vi "DataEmulator.vi"(1 "Time":u32, 2 "queue out":refnum<queue>) -> ()   [LabVIEW 2018]
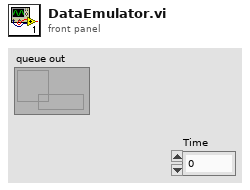
[diagram p1: front panel]
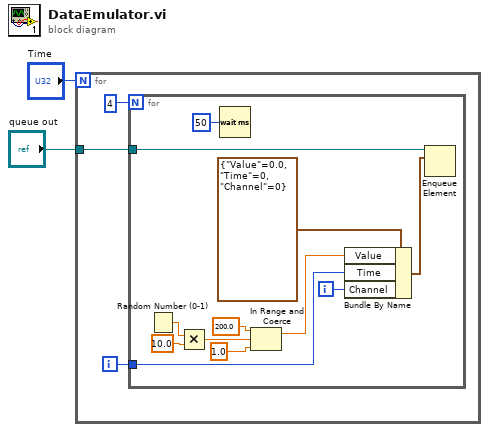
[diagram p0: block diagram]
diagram:
  n1 = for {
    N: "Time" -> [_]
    tunnel: "queue out" -> [w5]
    i -> [w4]
    n2 = for {
      N: 4 -> [_]
      tunnel: w5 -> [w17]
      tunnel: w4 -> [w7]
      i -> [w8]
      n3 = Random Number (0-1)() -> (number: 0 to 1=w16:dbl)
      n4 = Multiply(x=w16, y=10.0) -> (x*y=w14:dbl)
      n5 = Wait (ms)(milliseconds to wait=u32 50) -> ()  [unwired: 1 out]
      n6 = In Range and Coerce(upper limit=200.0, x=w14, lower limit=1.0) -> (coerced(x)=w9:dbl)  [unwired: 1 out]
      n7 = Bundle By Name(cluster=cluster{"Value":dbl, "Time":u32, "Channel":i32} {"Value"=0.0, "Time"=0, "Channel"=0}, "Value"=w9, "Time"=w7, "Channel"=w8) -> (w10:cluster{"Value":dbl, "Time":u32, "Channel":i32})
      n8 = Enqueue Element(queue=w17, element=w10) -> ()  [unwired: 2 in, 3 out]
    }
  }
